vi "ValidateFileAppenderConfigDTO.vi"(8 "error in (no error)":errorcluster, 11 "FileAppenderConfigDTOin":T1={"common"={"id"="", "threshold"="INFO", "filter"={"mode"="Mirror", "levelMin"="INFO", "levelMax"="INFO", "tagPrefix"=""}, "queueBound"=0, "dropPolicy"="DropOldest", "useUTC"=FALSE}, "file"={"rootFolder"="", "maxFileSize"=0, "maxFileCount"=0, "baseName"="", "extension"="", "delimiter"="", "calendarFolderTree"=FALSE}}) -> (0 "error out":errorcluster, 3 "FileAppenderConfigDTOout":T1={"common"={"id"="", "threshold"="INFO", "filter"={"mode"="mirror", "levelMin"="INFO", "levelMax"="INFO", "tagPrefix"=""}, "queueBound"=0, "dropPolicy"="dropOldest", "useUTC"=FALSE}, "file"={"rootFolder"="", "maxFileSize"=0, "maxFileCount"=0, "baseName"="", "extension"="", "delimiter"="", "calendarFolderTree"=FALSE}})   [LabVIEW 2026, in "Lumberjack.lvlib"]
uses:
  Lumberjack.lvlib
  <vilib>/Utility/Data Type/NI_Data Type.lvlib
  TypeDefs/ConfigDTO/FilterDTO.ctl
  TypeDefs/ConfigDTO/AppenderConfigDTO.ctl
  TypeDefs/ConfigDTO/FileConfigDTO.ctl
  TypeDefs/ConfigDTO/FileAppenderConfigDTO.ctl
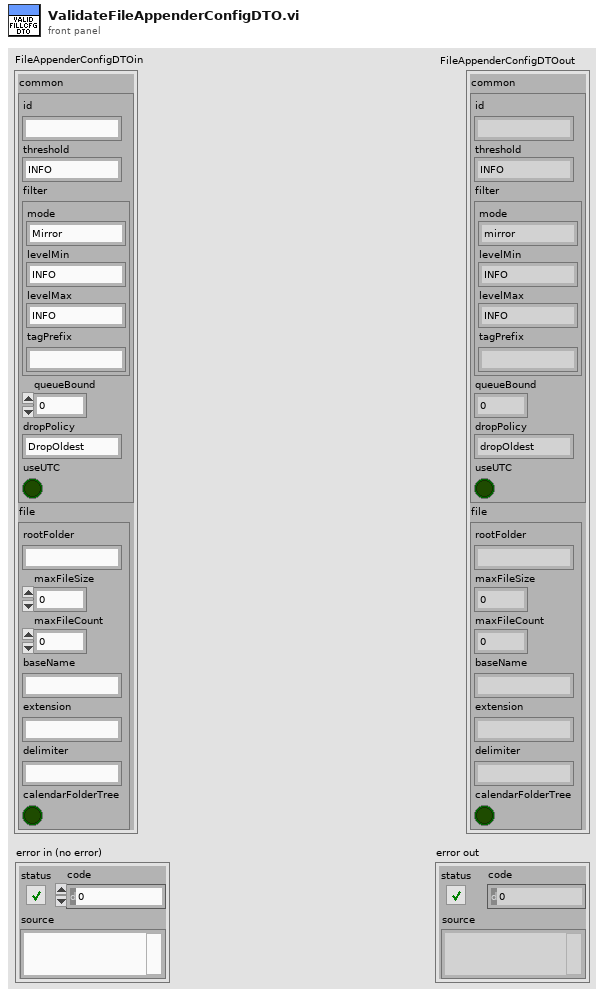
[diagram p1: front panel]
types:
  T1 = typedef "Lumberjack.lvlib/FileAppenderConfigDTO.ctl" = cluster{"common":T2, "file":T4}
  T2 = typedef "Lumberjack.lvlib/AppenderConfigDTO.ctl" = cluster{"id":string, "threshold":string, "filter":T3, "queueBound":i32, "dropPolicy":string, "useUTC":bool}
  T3 = typedef "Lumberjack.lvlib/FilterDTO.ctl" = cluster{"mode":string, "levelMin":string, "levelMax":string, "tagPrefix":string}
  T4 = typedef "Lumberjack.lvlib/FileConfigDTO.ctl" = cluster{"rootFolder":string, "maxFileSize":i64, "maxFileCount":i32, "baseName":string, "extension":string, "delimiter":string, "calendarFolderTree":bool}
  T5 = typedef "NI_Data Type.lvlib/Data Type.ctl" = enum8{"Invalid Type", "Void", "I8", "I16", "I32", "I64", "U8", "U16", "U32", "U64", "Single Float", "Double Float", "Extended Float", "Single Complex", "Double Complex", "Extended Complex", "Enum U8", "Enum U16", "Enum U32", "Enum U64", "Single Float With Unit", "Double Float With Unit", "Extended Float With Unit", "Single Complex with Unit", "Double Complex with Unit", "Extended Complex with Unit", "Boolean", "String", "Path", "Picture", "Tag", "Array", "Cluster", "Variant", "LV Variant", "Waveform", "Timestamp", "Digital Waveform", "Digital Data", "ExpressData", "Refnum", "External Data", "VI", "Poly VI", "LabVIEW Class Instance", "Fixed Point", "Set Collection", "Map Collection"}
  T6 = typedef "NI_Data Type.lvlib/Type Definition Info.ctl" = cluster{"Name":string, "Timestamp":u32}
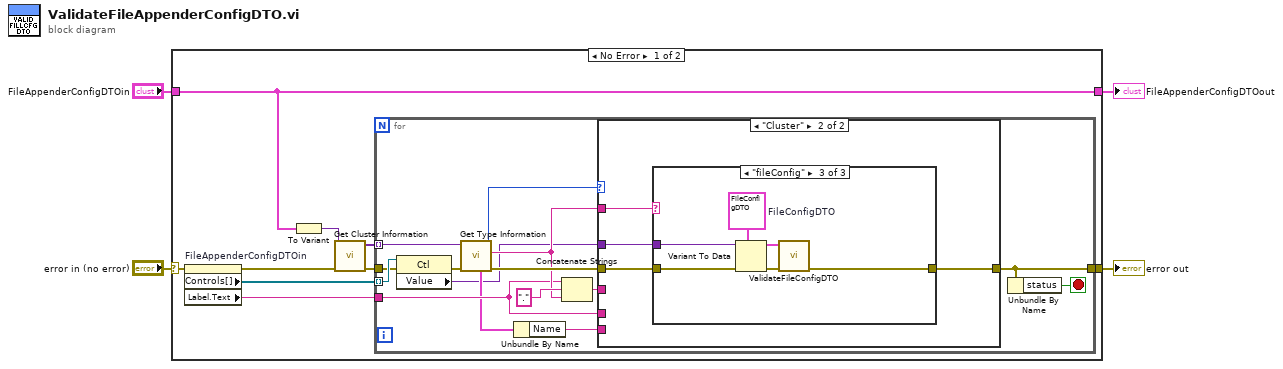
[diagram p0: block diagram]
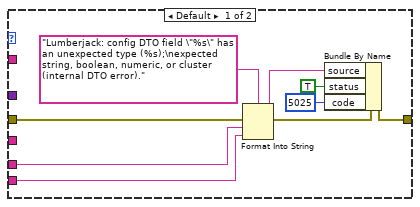
[diagram p2: hidden frame]
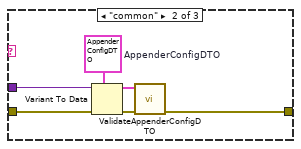
[diagram p4: hidden frame]
diagram:
  n1 = case shown="No Error" "error in (no error)" {
    selector: "error in (no error)" -> [w6 w55]
    tunnel: [w7 w55] -> w4
    tunnel: "FileAppenderConfigDTOin" -> [w5 w56]
    tunnel: [w5 w56] -> w1
    frame No Error {
      n2 = property on="FileAppenderConfigDTOin" class="Clust (strict)"(error in=w6) -> (error out=w11:errorcluster, "Controls[]"=w8:refnum<vi>[], "Label.Text"=w9:string)  [unwired: 1 in, 1 out]
      n3 = To Variant(anything=w5) -> (Variant=w10:variant)
      n4 = call <vilib>:"Get Cluster Information.vi"("error in (no error)"=w11, "variant"=w10) -> ("error out"=w12:errorcluster, "cluster elements"=w13:variant[])  [unwired: 8 in]
      n5 = for {
        tunnel: w13 -> [w23] mode=indexing
        tunnel: w12 -> [w16]
        tunnel: w9 -> [w22]
        tunnel: [w19] -> w7
        tunnel: w8 -> [w17] mode=indexing
        stop <- w18 stop-if-true
        n6 = property class="Ctl"(reference=w17, error in=w16) -> (error out=w14:errorcluster, "Value"=w15:variant)  [unwired: 1 out]
        n7 = call <vilib>:"Get Type Information.vi"("error in (no error)"=w14, "variant"=w23) -> ("error out"=w27:errorcluster, "name"=w24:string, "type"=w25:T5, "type definition info"=w21:T6)  [unwired: 5 in, 1 out]
        n8 = Unbundle By Name(w21) -> ("Name"=w20:string)
        n9 = Concatenate Strings(w22, "." ("string"), w24) -> (w26:string)
        n10 = case shown="\"Cluster\"" w25 {
          tunnel: w27 -> [w33 w41]
          tunnel: w26 -> [_ _]
          tunnel: w24 -> [_ w39]
          tunnel: w15 -> [_ w40]
          tunnel: w22 -> [w34 _]
          tunnel: [w30 w38] -> w19
          tunnel: w20 -> [w31 _]
          frame Default {
            n11 = Format Into String(format string="Lumberjack: config DTO field \"%s\" has an unexpected type (%s);\nexpected string, boolean, numeric, or cluster (internal DTO error)." ("source"), error in=w33, w34, w31) -> (resulting string=w29:string, error out=w32:errorcluster)  [unwired: 1 in]
            n12 = Bundle By Name(cluster=w32, "source"=w29, "status"=TRUE, "code"=5025) -> (w30:errorcluster)
          }
          frame "Cluster" {
            n13 = case shown="\"fileConfig\"" w39 {
              tunnel: w41 -> [w42 w48 w54]
              tunnel: w40 -> [_ w47 w53]
              tunnel: [w42 w44 w50] -> w38
              frame Default {
              }
              frame "common" {
                w43 = T2 {"id"="mirror", "threshold"="INFO", "filter"={"mode"="Mirror", "levelMin"="INFO", "levelMax"="INFO", "tagPrefix"=""}, "queueBound"=0, "dropPolicy"="DropOldest", "useUTC"=FALSE}  # AppenderConfigDTO
                n14 = Variant To Data(error in=w48, type=w43, Variant=w47) -> (data=w45:T2, error out=w46:errorcluster)
                n15 = call "ValidateAppenderConfigDTO.vi"("error in (no error)"=w46, "AppenderConfigDTOin"=w45) -> ("error out"=w44:errorcluster)  [unwired: 8 in, 1 out]
              }
              frame "fileConfig" {
                w49 = T4 {"rootFolder"="mirror", "maxFileSize"=0, "maxFileCount"=0, "baseName"="", "extension"="DropOldest", "delimiter"="", "calendarFolderTree"=FALSE}  # FileConfigDTO
                n16 = Variant To Data(error in=w54, type=w49, Variant=w53) -> (data=w51:T4, error out=w52:errorcluster)
                n17 = call "ValidateFileConfigDTO.vi"("error in (no error)"=w52, "FileConfigDTOin"=w51) -> ("error out"=w50:errorcluster)  [unwired: 8 in, 1 out]
              }
            }
          }
        }
        n18 = Unbundle By Name(w19) -> ("status"=w18:bool)
      }
    }
    frame Error {
    }
  }
  "error out" <- w4
  "FileAppenderConfigDTOout" <- w1
